vi "SimpleSweep_K2400 (rev1).vi"(4 "error in":errorcluster, 6 "SweepSettings":T1 {"Vstep (V)" format="%.3f"; "Vstop (V)" format="%.3f"; "Vstart (V)" format="%.3f"}) -> (0 "error out":errorcluster, 2 "XY Graph":cluster{dbl[], dbl[]}(graph), 3 "Result (V - I)":dbl[][](array[numeric]) format="%^#.6e")   [LabVIEW 2017]
uses:
  <vilib>/Utility/file.llb/Write To Spreadsheet File (DBL).vi
panel:
  out "t (s)":dbl
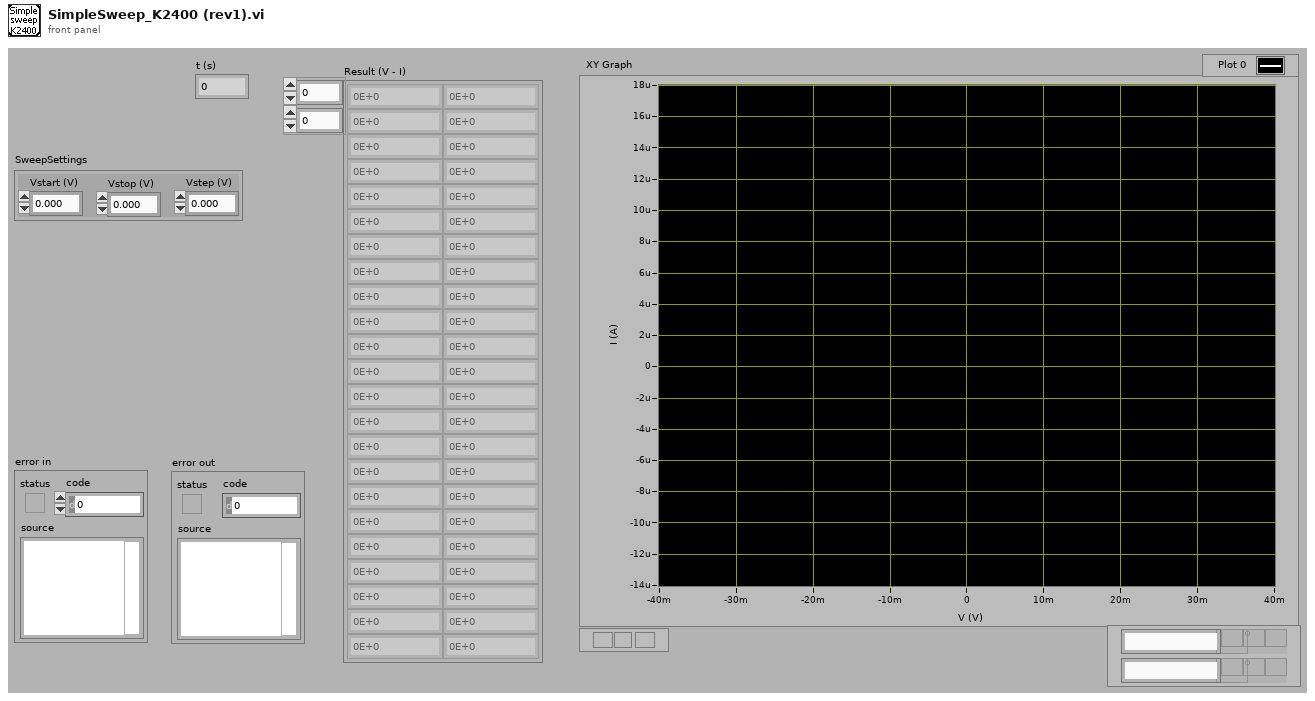
[diagram p1: front panel]
types:
  T1 = cluster{"Vstart (V)":dbl, "Vstop (V)":dbl, "Vstep (V)":dbl}
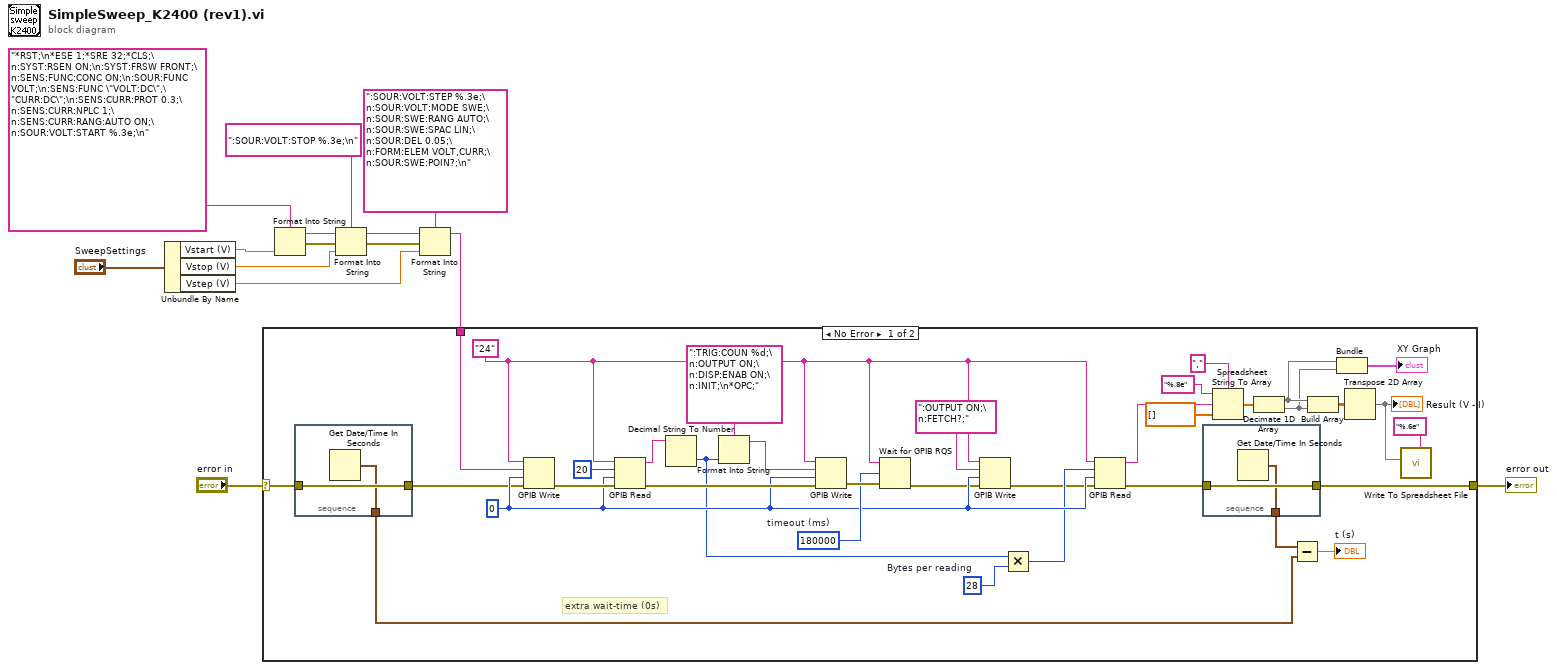
[diagram p0: block diagram]
diagram:
  n1 = Unbundle By Name("SweepSettings") -> ("Vstart (V)"=w5:dbl, "Vstop (V)"=w6:dbl, "Vstep (V)"=w4:dbl)
  n2 = Format Into String(format string="*RST;\n*ESE 1;*SRE 32;*CLS;\n:SYST:RSEN ON;\n:SYST:FRSW FRONT;\n:SENS:FUNC:CONC ON;\n:SOUR:FUNC VOLT;\n:SENS:FUNC \"VOLT:DC\",\"CURR:DC\";\n:SENS:CURR:PROT 0.3;\n:SENS:CURR:NPLC 1;\n:SENS:CURR:RANG:AUTO ON;\n:SOUR:VOLT:START %.3e;\n", w5) -> (resulting string=w12:string, error out=w10:errorcluster)  [unwired: 2 in]
  n3 = Format Into String(format string=":SOUR:VOLT:STOP %.3e;\n", initial string=w12, error in=w10, w6) -> (resulting string=w9:string, error out=w7:errorcluster)
  n4 = Format Into String(format string=":SOUR:VOLT:STEP %.3e;\n:SOUR:VOLT:MODE SWE;\n:SOUR:SWE:RANG AUTO;\n:SOUR:SWE:SPAC LIN;\n:SOUR:DEL 0.05;\n:FORM:ELEM VOLT,CURR;\n:SOUR:SWE:POIN?;\n", initial string=w9, error in=w7, w4) -> (resulting string=w1:string)  [unwired: 1 out]
  n5 = case shown="No Error" "error in" {
    selector: "error in" -> [w26 w54]
    tunnel: w1 -> [w43 _]
    tunnel: [w23 w54] -> w3
    frame No Error {
      w17 = "24" ("address string")
      w32 = i16 0 ("mode (0)")
      w30 = 28  # Bytes per reading
      w34 = 180000  # timeout (ms)
      # "extra wait-time (0s)"
      n6 = stacked-sequence {
        tunnel: w26 -> [w53]
        tunnel: [w53] -> w25
        tunnel: [w52] -> w21
        frame #0 {
          n7 = Get Date/Time In Seconds() -> (seconds since 1Jan1904=w52:timestamp)
        }
      }
      n8 = GPIB Write(0:w17, 1:w43, 2:w32, 3:w25) -> (6:w40:errorcluster)  [unwired: 1 in, 1 out]
      n9 = GPIB Read(0:w17, 1:20 ("byte count"), 2:w32, 3:w40) -> (5:w37:string, 7:w36:errorcluster)  [unwired: 1 in, 1 out]
      n10 = Decimal String To Number(string=w37) -> (number=w31:i32)  [unwired: 2 in, 1 out]
      n11 = Format Into String(format string=":TRIG:COUN %d;\n:OUTPUT ON;\n:DISP:ENAB ON;\n:INIT;\n*OPC;", w31) -> (resulting string=w38:string)  [unwired: 2 in, 1 out]
      n12 = GPIB Write(0:w17, 1:w38, 2:w32, 3:w36) -> (6:w35:errorcluster)  [unwired: 1 in, 1 out]
      n13 = Wait for GPIB RQS(2:w35, 3:w34, 4:w17) -> (0:w28:errorcluster)  [unwired: 1 out]
      n14 = GPIB Write(0:w17, 1:":OUTPUT ON;\n:FETCH?;", 2:w32, 3:w28) -> (6:w27:errorcluster)  [unwired: 1 in, 1 out]
      n15 = Multiply(x=w31, y=w30) -> (x*y=w29:i32)
      n16 = GPIB Read(0:w17, 1:w29, 2:w32, 3:w27) -> (5:w42:string, 7:w24:errorcluster)  [unwired: 1 in, 1 out]
      n17 = stacked-sequence {
        tunnel: w24 -> [w51]
        tunnel: [w51] -> w23
        tunnel: [w50] -> w22
        frame #0 {
          n18 = Get Date/Time In Seconds() -> (seconds since 1Jan1904=w50:timestamp)
        }
      }
      n19 = Spreadsheet String To Array(delimiter (Tab)=",", format string="%.8e", spreadsheet string=w42, array type (2D Dbl)=dbl[] []) -> (array=w46:dbl[])
      n20 = Decimate 1D Array(w46) -> (w19:dbl[], w18:dbl[])
      n21 = Subtract(x=w22, y=w21) -> (x-y=→"t (s)":dbl)
      n22 = Build Array(w19, w18) -> (w45:dbl[][])
      n23 = Bundle(w19, w18) -> (→"XY Graph":cluster{dbl[], dbl[]})  [unwired: 1 in]
      n24 = Transpose 2D Array(2D array=w45) -> (transposed array=w16:dbl[][])
      "Result (V - I)" <- w16
      n25 = call-poly <vilib>:"Write To Spreadsheet File.vi"("format (%.3f)"="%.6e", "2D data"=w16) -> ()  [unwired: 6 in, 1 out]
    }
    frame Error {
    }
  }
  "error out" <- w3
